vi "SerialNo.vi"() -> (2 "Continue?":bool)   [LabVIEW 2018]
uses:
  globals/QC_RunInformation.vi
panel:
  in  "DB Serial No.:":string
  in  "Batch No.:":string
  in  "Device Category:":string(combo)="ATLAS18SS"
  in  "Manufacturer:":string(combo)="Hamamatsu"
  in  "Sensor Serial No.:":string
  in  "Cancel":bool
  in  "OK":bool
  in  "Barcode reader":bool
  # "ATLAS Serial No."
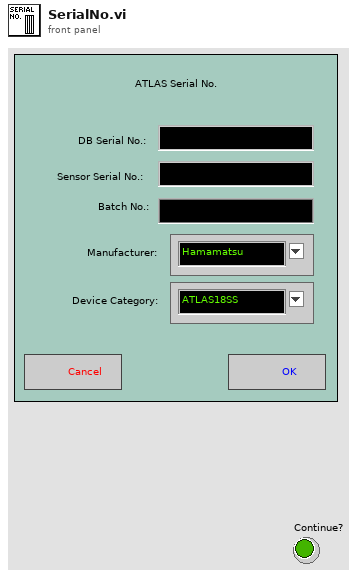
[diagram p1: front panel]
types:
  T1 = cluster{"Institute":string, "Manufacturers":string[], "Devices":string[], "Serialnumbers Lookup DB":string, "Data directory":string, "Backup & screenshot directory":string, "List of known users":string[]}
  T2 = cluster{"Sensor Serial No.:":string, "Wafer Serial No.:":string, "Batch:":string, "Manufacturer:":string, "Device Category:":string, "Database Serial No.:":string, "Date Initiated:":string, "Time Initiated:":string, "Test":string, "Instruments used:":string, "Probeplan used:":string, "End of Run comment:":string, "User:":string}
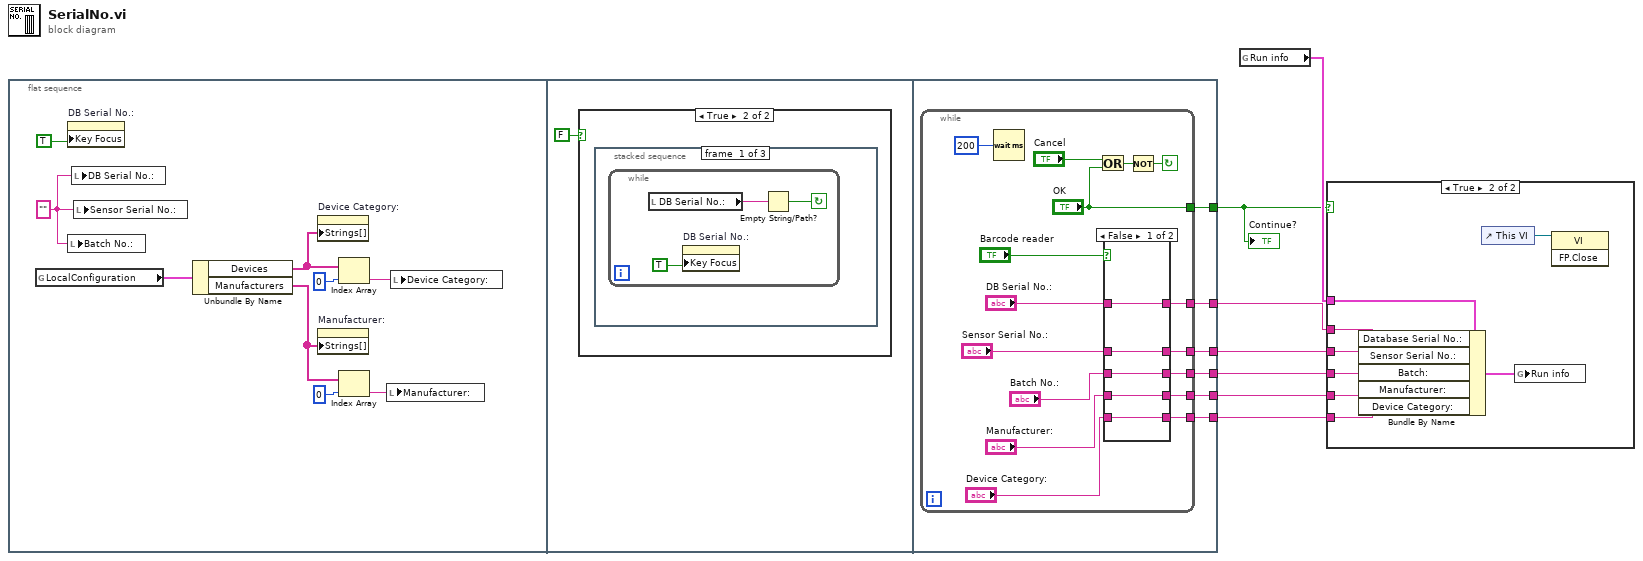
[diagram p0: block diagram]
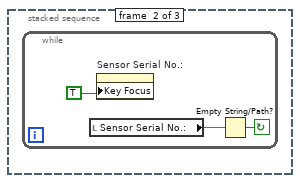
[diagram p4: hidden frame]
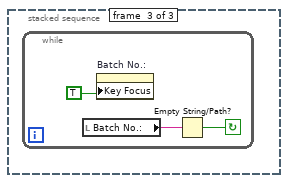
[diagram p5: hidden frame]
diagram:
  n1 = flat-sequence {
    tunnel: [w32] -> w7
    tunnel: [w31] -> w2
    tunnel: [w30] -> w5
    tunnel: [w29] -> w6
    tunnel: [w28] -> w1
    tunnel: [w27] -> w3
    frame #0 {
      w16 = ""
      n2 = global read "QC_RunInformation.vi" "LocalConfiguration"() -> (w14:T1)
      n3 = property on="DB Serial No.:" class="Str"("Key Focus"=TRUE) -> ()  [unwired: 2 in, 2 out]
      n4 = local write "Batch No.:"(w16) -> ()
      n5 = local write "DB Serial No.:"(w16) -> ()
      n6 = local write "Sensor Serial No.:"(w16) -> ()
      n7 = Unbundle By Name(w14) -> ("Devices"=w9:string[], "Manufacturers"=w8:string[])
      n8 = property on="Device Category:" class="CmbBox"("Strings[]"=w9) -> ()  [unwired: 2 in, 2 out]
      n9 = property on="Manufacturer:" class="CmbBox"("Strings[]"=w8) -> ()  [unwired: 2 in, 2 out]
      n10 = Index Array(array=w9, index=0) -> (element=w10:string)
      n11 = Index Array(array=w8, index=0) -> (element=w11:string)
      n12 = local write "Manufacturer:"(w11) -> ()
      n13 = local write "Device Category:"(w10) -> ()
    }
    frame #1 {
      n14 = case shown="True" FALSE {
        frame False {
        }
        frame True {
          n15 = stacked-sequence {
            frame #0 {
              n16 = while {
                stop <- w18 continue-if-true
                n17 = local read "DB Serial No.:"() -> (w19:string)
                n18 = property on="DB Serial No.:" class="Str"("Key Focus"=TRUE) -> ()  [unwired: 2 in, 2 out]
                n19 = Empty String/Path?(string/path=w19) -> (empty?=w18:bool)
              }
            }
            frame #1 {
              n20 = while {
                stop <- w22 continue-if-true
                n21 = local read "Sensor Serial No.:"() -> (w21:string)
                n22 = property on="Sensor Serial No.:" class="Str"("Key Focus"=TRUE) -> ()  [unwired: 2 in, 2 out]
                n23 = Empty String/Path?(string/path=w21) -> (empty?=w22:bool)
              }
            }
            frame #2 {
              n24 = while {
                stop <- w25 continue-if-true
                n25 = local read "Batch No.:"() -> (w24:string)
                n26 = property on="Batch No.:" class="Str"("Key Focus"=TRUE) -> ()  [unwired: 2 in, 2 out]
                n27 = Empty String/Path?(string/path=w24) -> (empty?=w25:bool)
              }
            }
          }
        }
      }
    }
    frame #2 {
      n28 = while {
        tunnel: ["OK"] -> w31
        tunnel: [w41] -> w28
        tunnel: [w42] -> w32
        tunnel: [w40] -> w27
        tunnel: [w39] -> w30
        tunnel: [w38] -> w29
        stop <- w46 continue-if-true
        n29 = Wait (ms)(milliseconds to wait=200) -> ()  [unwired: 1 out]
        n30 = Or(x="Cancel", y="OK") -> (x .or. y?=w47:bool)
        n31 = case shown="False" "Barcode reader" {
          tunnel: "DB Serial No.:" -> [w53 w58]
          tunnel: "Sensor Serial No.:" -> [w52 w57]
          tunnel: [w53 w58] -> w42
          tunnel: [w52 w57] -> w41
          tunnel: "Batch No.:" -> [w51 w56]
          tunnel: [w51 w56] -> w40
          tunnel: "Manufacturer:" -> [w50 w55]
          tunnel: [w50 w55] -> w39
          tunnel: "Device Category:" -> [w49 w54]
          tunnel: [w49 w54] -> w38
          frame False {
          }
          frame True {
          }
        }
        n32 = Not(x=w47) -> (.not. x?=w46:bool)
      }
    }
  }
  n33 = global read "QC_RunInformation.vi" "Run info"() -> (w4:T2)
  n34 = case shown="True" w2 {
    tunnel: w7 -> [_ w66]
    tunnel: w6 -> [_ w65]
    tunnel: w5 -> [_ w64]
    tunnel: w4 -> [_ w63]
    tunnel: w3 -> [_ w62]
    tunnel: w1 -> [_ w60]
    frame False {
    }
    frame True {
      n35 = Bundle By Name(cluster=w63, "Database Serial No.:"=w66, "Sensor Serial No.:"=w60, "Batch:"=w62, "Manufacturer:"=w64, "Device Category:"=w65) -> (w61:T2)
      n36 = control-ref of="This VI"() -> (w59:refnum<vi>)
      n37 = global write "QC_RunInformation.vi" "Run info"(w61) -> ()
      n38 = invoke class="VI" method="FP.Close"(reference=w59) -> ()  [unwired: 2 in, 3 out]
    }
  }
  "Continue?" <- w2
